vi "CheckFileExist_theirs.vi"(7 "format string":string="%03d", 8 "error in (no error) 2":errorcluster, 9 "Path separator (\\)":string="\\", 10 "Interactive":bool=TRUE, 11 "File in":path) -> (0 "error out":errorcluster, 2 "Overwrite":bool, 3 "File out":path)   [LabVIEW 2015]
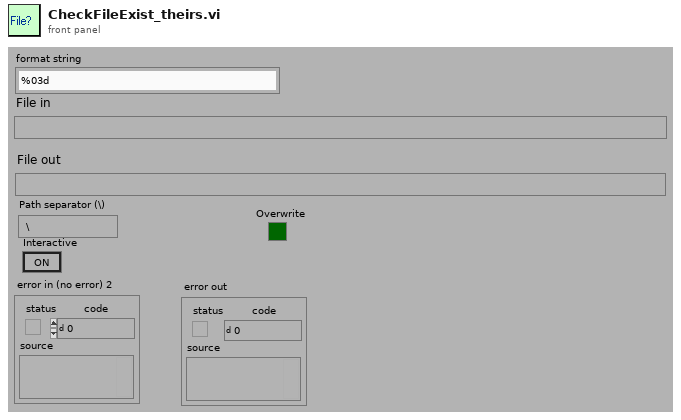
[diagram p1: front panel]
types:
  T1 = enum32{"existing file", "new file", "new or existing file", "existing dir", "new dir", "new or existing dir", "existing file (use LLBs)", "new file (use LLBs)", "new or existing file (use LLBs)", "new or existing file or directory (use LLBs)", "existing dir (use LLBs)", "new dir (use LLBs)", "new or existing dir (use LLBs)", "existing file or dir", "new file or dir", "new or existing file or dir", "existing file or dir (use LLBs)", "new file or dir (use LLBs)"}
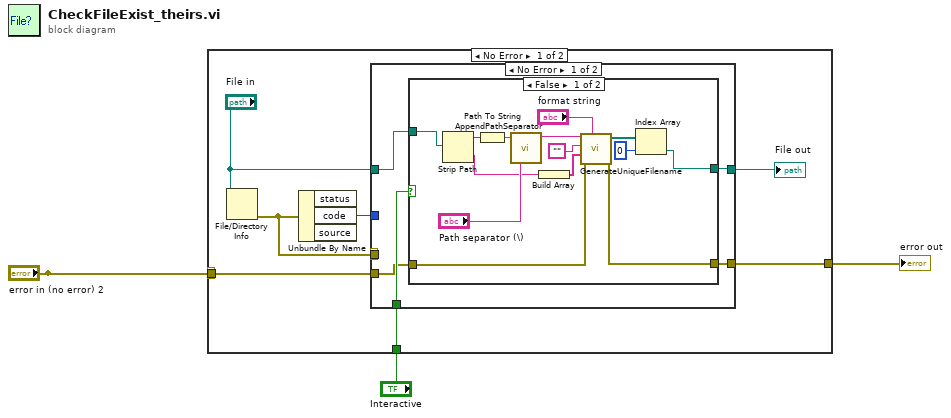
[diagram p0: block diagram]
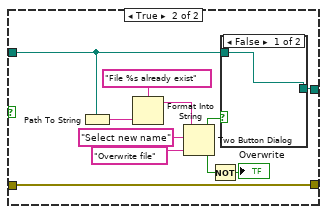
[diagram p2: hidden frame]
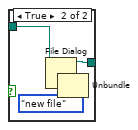
[diagram p3: hidden frame]
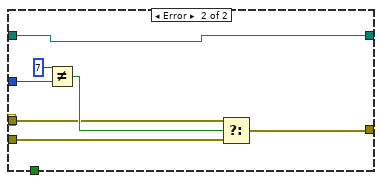
[diagram p4: hidden frame]
diagram:
  n1 = case shown="No Error" "error in (no error) 2" {
    tunnel: "Interactive" -> [w7 _]
    tunnel: [w5 w51] -> w2
    tunnel: "error in (no error) 2" -> [w6 w51]
    frame No Error {
      n2 = File/Directory Info(path="File in") -> (error out=w4:errorcluster)  [unwired: 1 in, 6 out]
      n3 = Unbundle By Name(w4) -> ("code"=w10:i32)  [unwired: 2 out]
      n4 = case shown="No Error" w4 {
        tunnel: w10 -> [_ w49]
        tunnel: "File in" -> [w14 w48]
        tunnel: w4 -> [_ w45]
        tunnel: [w15 w48] -> w8
        tunnel: w7 -> [w13 _]
        tunnel: w6 -> [w12 w44]
        tunnel: [w11 w47] -> w5
        frame No Error {
          n5 = case shown="False" w13 {
            tunnel: [w19 w39] -> w15
            tunnel: w14 -> [w29 w35]
            tunnel: w12 -> [w24 w31]
            tunnel: [w23 w31] -> w11
            frame False {
              n6 = Strip Path(path=w29) -> (stripped path=w28:path, name=w25:string)
              n7 = Path To String(path=w28) -> (string=w27:string)
              n8 = call "AppendPathSeparator.vi"("Path separator (\\)"="Path separator (\\)", "Path"=w27) -> ("Dup path with separator"=w16:string)  [unwired: 9 out]
              n9 = Build Array(w25) -> (w21:string[])
              n10 = call "GenerateUniqueFilename.vi"("format string"="format string", "error in (no error)"=w24, "File Name Suffixes"=w21, "File Name Prefix"="", "Folder"=w16) -> ("error out"=w23:errorcluster, "Paths"=w22:path[])  [unwired: 5 out]
              n11 = Index Array(array=w22, index=0) -> (element=w19:path)
            }
            frame True {
              n12 = Path To String(path=w35) -> (string=w34:string)
              n13 = Format Into String(format string="File %s already exist", w34) -> (resulting string=w32:string)  [unwired: 2 in, 1 out]
              n14 = Two Button Dialog(message=w32, 1:"Overwrite file", 2:"Select new name") -> (T button?=w36:bool)
              n15 = Not(x=w36) -> (.not. x?=→"Overwrite":bool)
              n16 = case shown="False" w36 {
                tunnel: [w40 w43] -> w39
                tunnel: w35 -> [w40 w42]
                frame False {
                }
                frame True {
                  (unwired) T1."new file" ("select mode (2)")
                  n17 = File Dialog(11:w42) -> (0:w41:errorcluster, 3:w43:path)  [unwired: 1 in, 7 out]
                  n18 = Unbundle(w41) -> ()  [unwired: 3 out]
                }
              }
            }
          }
        }
        frame Error {
          n19 = Not Equal?(x=7, y=w49) -> (x != y?=w46:bool)
          n20 = Select(t=w45, s=w46, f=w44) -> (s? t:f=w47:errorcluster)
        }
      }
      "File out" <- w8
    }
    frame Error {
    }
  }
  "error out" <- w2
